vi "Gerador de sinais.vi"() -> ()   [LabVIEW 2019]
uses:
  Estados.ctl
  <vilib>/measure/NI_MABase.lvlib
panel:
  out "Waveform Graph":waveform(dbl)(graph)
  in  "offset":dbl format="%.2p"
  in  "phase":dbl format="%.2p"
  in  "amplitude":dbl=1.0 format="%.2p"
  in  "frequency":dbl=10.0 format="%.2p"
  in  "?":T1
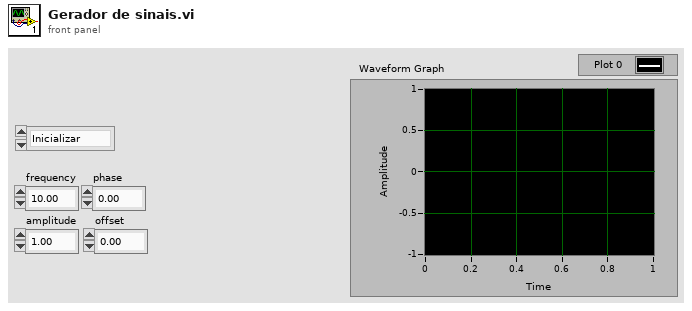
[diagram p1: front panel]
types:
  T1 = typedef "Estados.ctl" = enum16{"Inicializar", "Esperar por evento", "Quadrada", "Senoidal", "Triangular", "Dente de Serra", "Trapezoidal"}
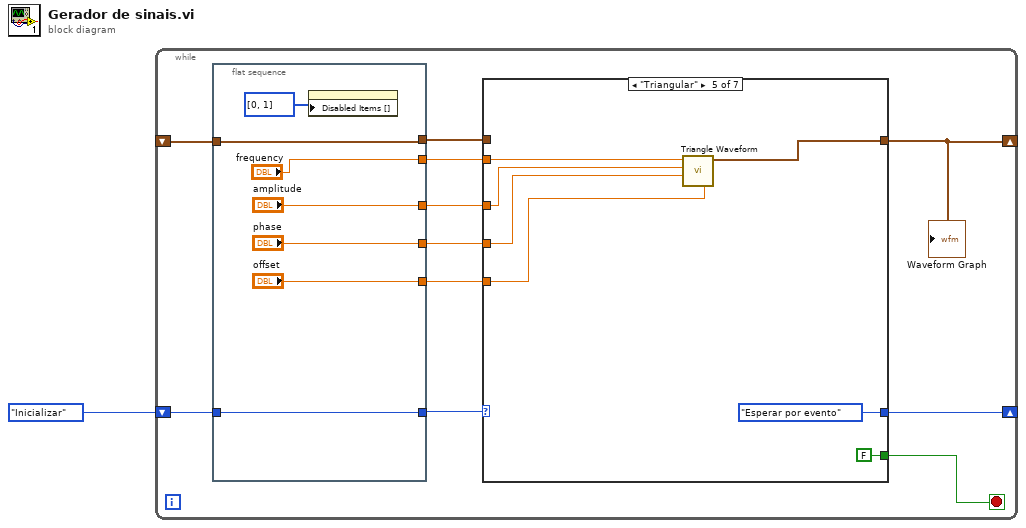
[diagram p0: block diagram]
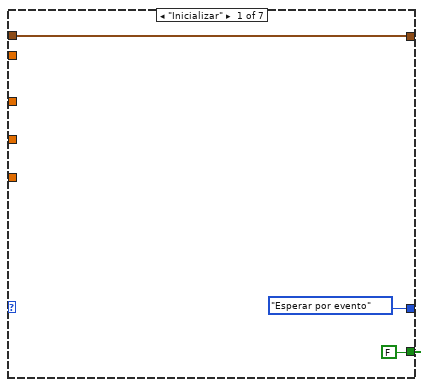
[diagram p2: hidden frame]
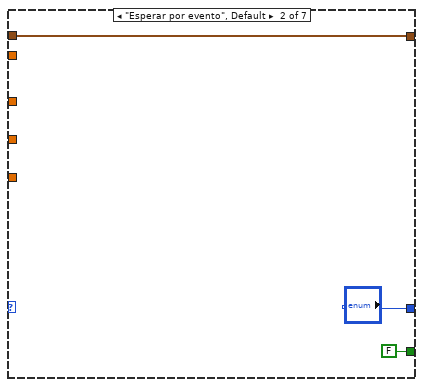
[diagram p3: hidden frame]
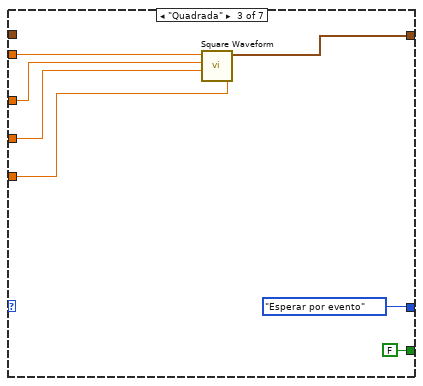
[diagram p4: hidden frame]
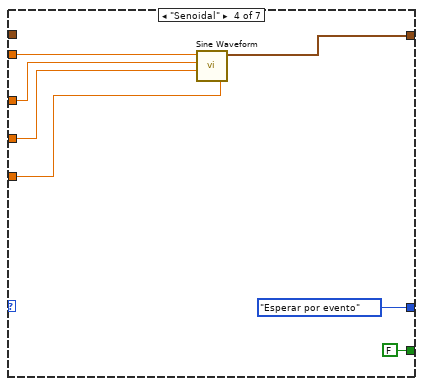
[diagram p5: hidden frame]
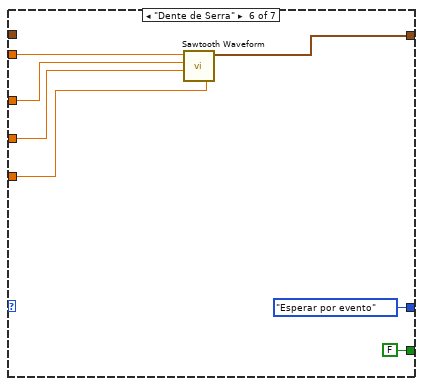
[diagram p6: hidden frame]
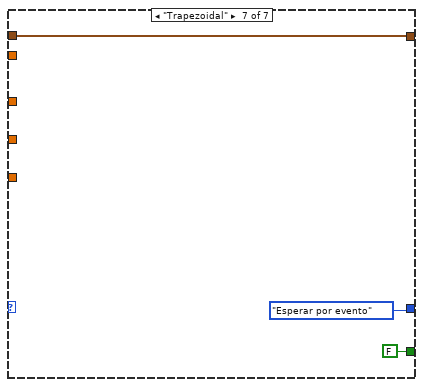
[diagram p7: hidden frame]
diagram:
  n1 = while {
    shift-right: [w12] -> _
    shift-left: Estados."Inicializar" -> [w5]
    shift-right: [w4] -> _
    shift-left: _ -> [w3]
    stop <- w11 stop-if-true
    n2 = flat-sequence {
      tunnel: ["frequency"] -> w10
      tunnel: ["amplitude"] -> w9
      tunnel: ["phase"] -> w8
      tunnel: ["offset"] -> w7
      tunnel: [w14] -> w6
      tunnel: w5 -> [w14]
      tunnel: [w13] -> w2
      tunnel: w3 -> [w13]
      frame #0 {
        n3 = property class="Enum (strict)"("Disabled Items []"=i32[] [0, 1]) -> ()  [unwired: 2 in, 2 out]
      }
    }
    n4 = case shown="\"Triangular\"" w6 {
      tunnel: [Estados."Esperar por evento" "?" Estados."Esperar por evento" Estados."Esperar por evento" Estados."Esperar por evento" Estados."Esperar por evento" Estados."Esperar por evento"] -> w12
      tunnel: [FALSE FALSE FALSE FALSE FALSE FALSE FALSE] -> w11
      tunnel: w10 -> [_ _ w29 w36 w43 w53 _]
      tunnel: w9 -> [_ _ w28 w35 w42 w52 _]
      tunnel: w8 -> [_ _ w27 w34 w41 w51 _]
      tunnel: w7 -> [_ _ w26 w33 w40 w50 _]
      tunnel: [w20 w23 w32 w39 w46 w49 w54] -> w4
      tunnel: w2 -> [w20 w23 _ _ _ _ w54]
      frame "Inicializar" {
      }
      frame "Esperar por evento", Default {
      }
      frame "Quadrada" {
        n5 = call <vilib>:"Square Waveform.vi"("offset"=w26, "phase"=w27, "amplitude"=w28, "frequency"=w29) -> ("signal out"=w32:waveform(dbl))  [unwired: 6 in, 1 out]
      }
      frame "Senoidal" {
        n6 = call <vilib>:"Sine Waveform.vi"("offset"=w33, "phase"=w34, "amplitude"=w35, "frequency"=w36) -> ("signal out"=w39:waveform(dbl))  [unwired: 6 in, 1 out]
      }
      frame "Triangular" {
        n7 = call <vilib>:"Triangle Waveform.vi"("offset"=w40, "phase"=w41, "amplitude"=w42, "frequency"=w43) -> ("signal out"=w46:waveform(dbl))  [unwired: 6 in, 1 out]
      }
      frame "Dente de Serra" {
        n8 = call <vilib>:"Sawtooth Waveform.vi"("offset"=w50, "phase"=w51, "amplitude"=w52, "frequency"=w53) -> ("signal out"=w49:waveform(dbl))  [unwired: 6 in, 1 out]
      }
      frame "Trapezoidal" {
      }
    }
    "Waveform Graph" <- w4
  }
